vi "read gain.vi"(0 "VISA resource name":refnum<visa-resource-name>="GPIB0::12::INSTR", 1 "error in (no error)":errorcluster) -> (2 "VISA resource name out":refnum<visa-resource-name>, 3 "Gain (%)":dbl, 4 "error out":errorcluster)   [LabVIEW 2015, in "MicrowaveAmplifier.lvlib"]
uses:
  MicrowaveAmplifier.lvlib
panel:
  out "read buffer":string
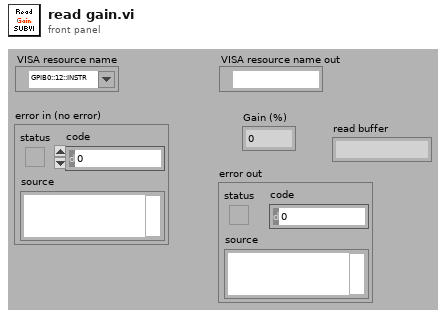
[diagram p1: front panel]
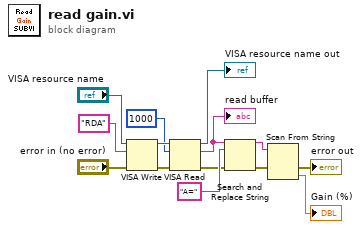
[diagram p0: block diagram]
diagram:
  n1 = VISA Write(VISA resource name="VISA resource name", write buffer="RDA", error in (no error)="error in (no error)") -> (VISA resource name out=w11:refnum<visa-resource-name>, error out=w12:errorcluster)  [unwired: 1 out]
  n2 = VISA Read(VISA resource name=w11, byte count=u32 1000, error in (no error)=w12) -> (VISA resource name out=→"VISA resource name out":refnum<visa-resource-name>, read buffer=w14:string, error out=w2:errorcluster)  [unwired: 1 out]
  "read buffer" <- w14
  n3 = Search and Replace String(input string=w14, search string="A=", error in=w2) -> (result string=w5:string, error out=w3:errorcluster)  [unwired: 5 in, 2 out]
  n4 = Scan From String(input string=w5, error in=w3) -> (error out=→"error out":errorcluster, output 1=→"Gain (%)":dbl)  [unwired: 3 in, 2 out]
